vi "Write Temperature Status.vi"(8 "error in (no error)":errorcluster, 10 "Temperature Status":T1, 11 "CCDCamera in":refnum<class "Simulated_CCD_Camera.lvclass">) -> (0 "error out":errorcluster, 3 "CCDCamera out":refnum<class "Simulated_CCD_Camera.lvclass">)   [LabVIEW 2018, in "Simulated_CCD_Camera.lvclass"]
uses:
  Simulated_CCD_Camera.lvclass
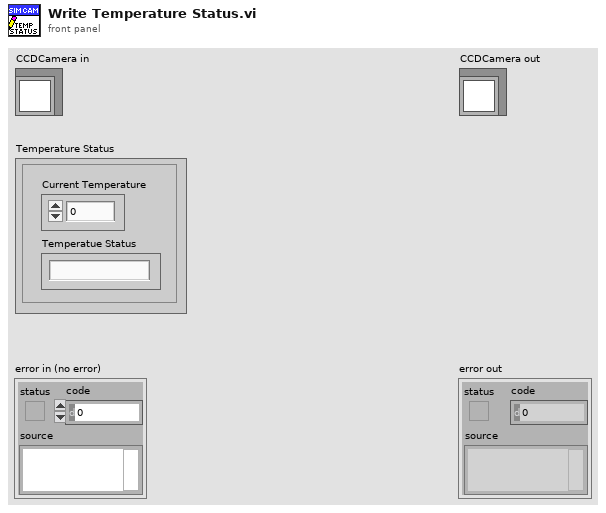
[diagram p1: front panel]
types:
  T1 = cluster{"Current Temperature":i32, "Temperatue Status":string}
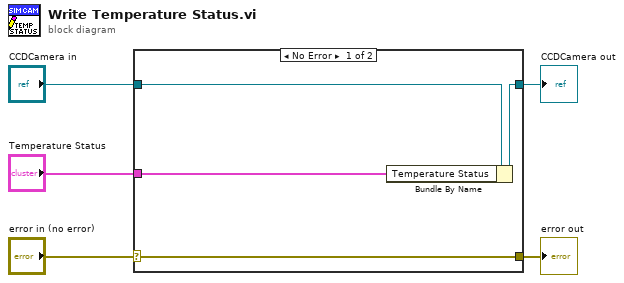
[diagram p0: block diagram]
diagram:
  n1 = case shown="No Error" "error in (no error)" {
    selector: "error in (no error)" -> [w9 w10]
    tunnel: [w9 w10] -> w4
    tunnel: [w7 w11] -> w2
    tunnel: "CCDCamera in" -> [w8 w11]
    tunnel: "Temperature Status" -> [w6 _]
    frame No Error {
      n2 = Bundle By Name(cluster=w8, "Temperature Status"=w6) -> (w7:refnum<class "Simulated_CCD_Camera.lvclass">)
    }
    frame Error {
    }
  }
  "error out" <- w4
  "CCDCamera out" <- w2
